vi "Alrebei.vi"() -> ()   [LabVIEW 2019]
panel:
  out "NH3/CH4":bool
  out "CH4":bool
  in  "Fuel Type":bool
  out "Waveform Chart":dbl(graph)
  out "time":dbl
  out "Controller":bool
  in  "PID gains":T1={"proportional gain (Kc)"=1.0, "integral time (Ti, min)"=0.01, "derivative time (Td, min)"=0.0} {"derivative time (Td, min)" format="%.3f"; "integral time (Ti, min)" format="%.3f"; "proportional gain (Kc)" format="%.3f"}
  in  "Fuel Control   (On/OFF)":bool=TRUE
  out "Controlled fuel\n       (kg/s)l":dbl
  out "Net Work (kW)":dbl(knob) scale=0.0..3000.0
  out "Turbine Work (kW)":dbl(knob) scale=0.0..3000.0
  out "Dilution Compressor Work (kW)":dbl(knob) scale=0.0..1000.0
  out "?":dbl(knob) scale=0.0..1000.0
  out "Dilution Compressor Work (kJ/Kg)":dbl(knob) scale=0.0..1000.0
  out "Flue gas  (kg/s)":dbl
  out "Comb. total (kg/s)":dbl(slide)
  out "?":dbl(slide) scale=0.0..2.5
  out "Comb. Air (kg/s)":dbl
  out "?":bool
  in  "Dilution Air (kg/s)":dbl(slide) scale=0.0..4.0
  out "?":bool
  out "?":bool
  out "?":bool
  out "?":bool
  out "Dilution Graphics.":bool
  out "?":dbl(slide)
  out "?":dbl(slide) scale=0.0..4.2
  out "Stoic. Condition":dbl
  out "?":dbl(slide)
  out "Comp. Air outlet Graphics":dbl(slide) scale=0.0..2.5
  out "?":dbl(slide)
  out "Fuel Graphics":dbl(slide) scale=0.0..0.14
  out "?":dbl(slide)
  out "?":dbl(slide) scale=0.0..0.14
  in  "Primery Air (kg/s)":dbl(slide) scale=1.0..4.0
  in  "Fuel (kg/s)":dbl(slide) scale=0.0..0.14
  out "?":dbl(slide)
  out "Primery Air  Graphics":dbl(slide) scale=0.0..4.0
  in  "Turbi. Eff.":dbl
  out "Turbine Outlet Prs.  (bar)":dbl(knob) scale=0.0..10.0
  out "Turbine Outlet Temp.  (K)":dbl(slide) scale=0.0..2000.0
  out "Turbine Work (kJ/kg)":dbl(knob) scale=0.0..3000.0
  out "Primery Compressor Work  (kJ/kg)      Primery Compressor Work ( kW)":dbl(knob) scale=0.0..1000.0
  in  "compressor \nefficiency":dbl
  out "ON/OFF":bool
  in  "RUN":bool
  out "Net Work (kJ/kg)":dbl(knob) scale=0.0..3000.0
  in  "Turbine Pres. ratio":dbl(slide) scale=0.0..1.0
  in  "Comp. Pres. ratio":dbl(slide) scale=0.0..10.0
  in  "Compressor\nTemp.":dbl(slide) scale=0.0..800.0
  in  "Compressor  Inlet Pressure  (bar)":dbl(knob) scale=0.0..3.0
  out "Turbine Inlet Temp. (K)":dbl(slide) scale=0.0..2000.0
  out "Turbine Inlet Pressure.\n               (bar)":dbl(knob) scale=0.0..10.0
  out "Compressor outlet Temp. (K)":dbl(slide) scale=0.0..1500.0
  out "Compressor outlet  pressure (bar)":dbl(knob) scale=0.0..10.0
  out "FUEL REDUCTION IS REQUIRED":bool
  out "DILUATION IS REQUIRED":bool
  out "Action Required":string
  out "COOLING IS ENOUGH":bool
  in  "Min T(K)":dbl
  in  "Max T (K)":dbl
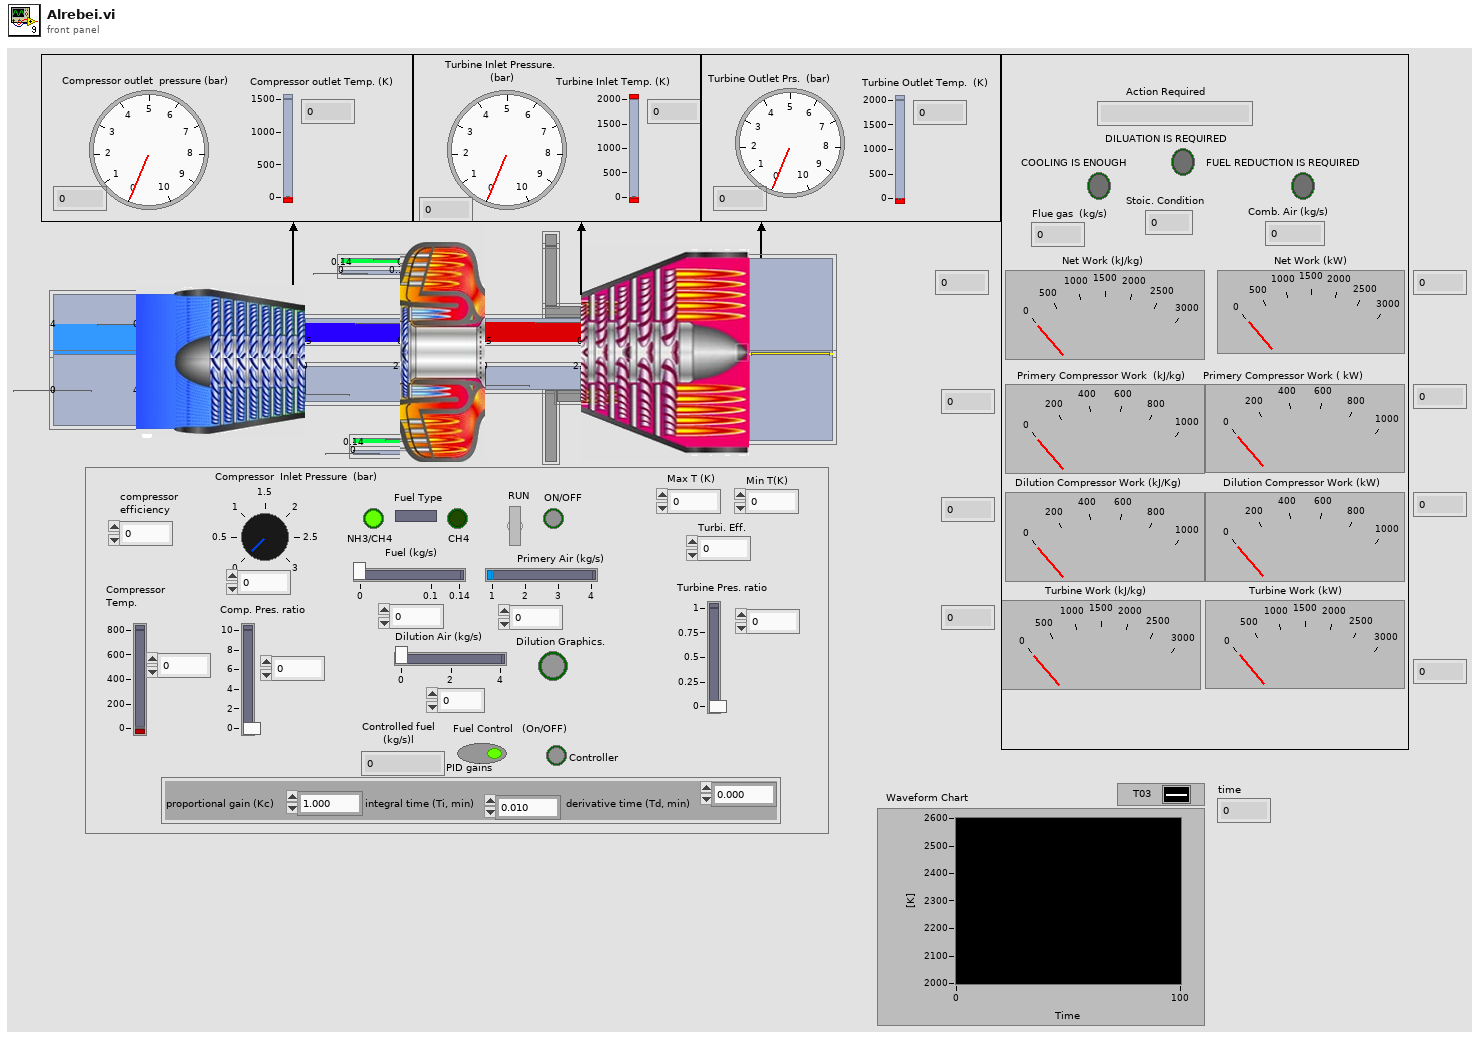
[diagram p1: front panel]
types:
  T1 = cluster{"proportional gain (Kc)":dbl, "integral time (Ti, min)":dbl, "derivative time (Td, min)":dbl}
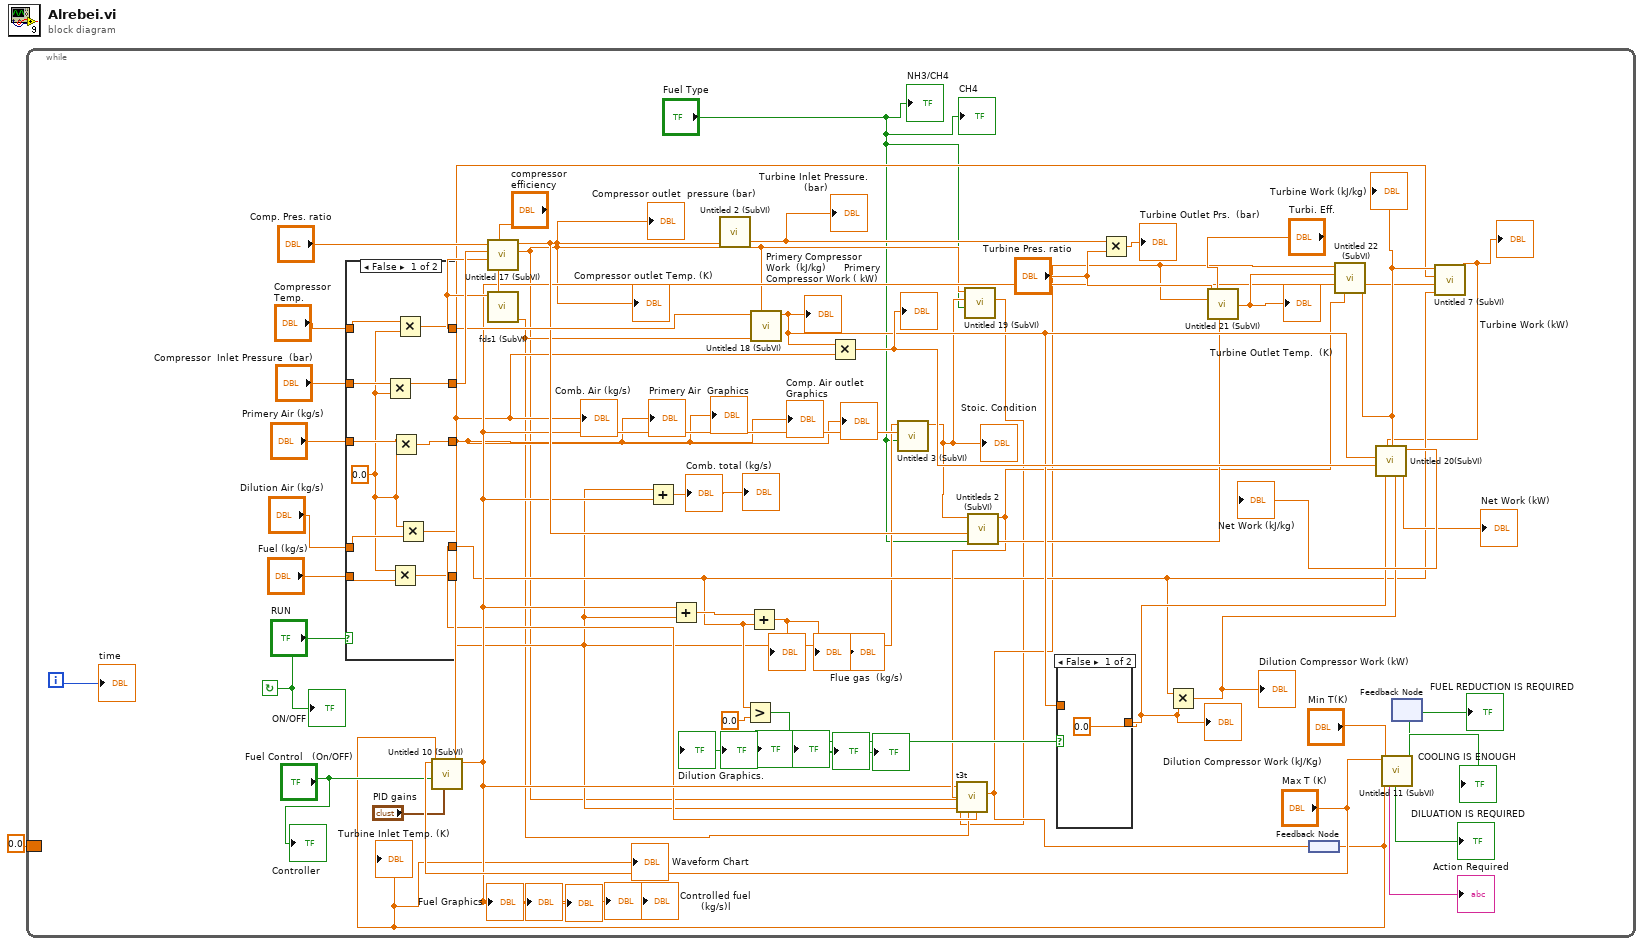
[diagram p0: block diagram]
diagram:
  n1 = while {
    border: 0.0 -> [_]
    i -> [w9]
    stop <- "RUN" continue-if-true
    n2 = case shown="False" "RUN" {
      tunnel: [w64 w71] -> w30
      tunnel: [w65 w72] -> w12
      tunnel: "Primery Air (kg/s)" -> [w67 w72]
      tunnel: "Fuel (kg/s)" -> [w66 w71]
      tunnel: [w62 w70] -> w13
      tunnel: "Dilution Air (kg/s)" -> [w63 w70]
      tunnel: [w60 w69] -> w39
      tunnel: "Compressor  Inlet Pressure  (bar)" -> [w61 w69]
      tunnel: [w58 w68] -> w21
      tunnel: "Compressor\nTemp." -> [w59 w68]
      frame False {
        w57 = 0.0
        n3 = Multiply(x=w61, y=w57) -> (x*y=w60:dbl)
        n4 = Multiply(x=w57, y=w66) -> (x*y=w64:dbl)
        n5 = Multiply(x=w67, y=w57) -> (x*y=w65:dbl)
        n6 = Multiply(x=w59, y=w57) -> (x*y=w58:dbl)
        n7 = Multiply(x=w57, y=w63) -> (x*y=w62:dbl)
      }
      frame True {
      }
    }
    "Primery Air  Graphics" <- w12
    "?" <- w12
    "Comp. Air outlet Graphics" <- w12
    "?" <- w12
    "Comb. Air (kg/s)" <- w12
    n8 = call "fds1 (SubVI).vi"("Compressor\nTemp."=w21) -> ("cpair"=w10:dbl, "gammair"=w20:dbl)  [unwired: 9 in]
    n9 = call "Untitled 17 (SubVI).vi"("Comp. Eff"="compressor \nefficiency", "gammaair"=w20, "Compressor inlet Tempreture (K)"=w21, "Compressor Inlet Pressure (bar)"=w39, "Compressor pressure ratio"="Comp. Pres. ratio") -> ("Compressor outlet Temp. (K)"=w6:dbl, "Compressor outlet Prs. (bar)"=w19:dbl)  [unwired: 5 in]
    "Compressor outlet  pressure (bar)" <- w19
    "Compressor outlet Temp. (K)" <- w6
    n10 = call "Untitled 2 (SubVI).vi"("Numeric in"=w19) -> ("Numeric out"=w48:dbl)  [unwired: 10 in]
    "Turbine Inlet Pressure.\n               (bar)" <- w48
    n11 = Greater?(x=w13, y=0.0) -> (0:w24:bool)
    "Dilution Graphics." <- w24
    "?" <- w24
    "?" <- w24
    "?" <- w24
    "?" <- w24
    "?" <- w24
    n12 = call "Untitled 18 (SubVI).vi"("Cpair"=w10, "Numeric in"=w6, "Compressor inlet Tempreture (K)"=w21) -> ("Numeric out"=w25:dbl)  [unwired: 8 in]
    "Primery Compressor Work  (kJ/kg)      Primery Compressor Work ( kW)" <- w25
    n13 = Multiply(x=w25, y=w12) -> (x*y=w33:dbl)
    "?" <- w33
    n14 = case shown="False" w24 {
      tunnel: w25 -> [_ w56]
      tunnel: [0.0 w56] -> w22
      frame False {
      }
      frame True {
      }
    }
    "Dilution Compressor Work (kJ/Kg)" <- w22
    n15 = Multiply(x=w48, y="Turbine Pres. ratio") -> (x*y=→"Turbine Outlet Prs.  (bar)":dbl)
    n16 = Multiply(x=w13, y=w22) -> (x*y=w34:dbl)
    "Dilution Compressor Work (kW)" <- w34
    n17 = feedback #1() -> (w8:dbl)
    "Turbine Inlet Temp. (K)" <- w8
    "Waveform Chart" <- w8
    n18 = call "Untitled 10 (SubVI).vi"("Fuel (kg/s)"=w30, "PID gains"="PID gains", "Fuel Control   (On/OFF)"="Fuel Control   (On/OFF)", "Numeric"=w8, "Max T (K)"="Max T (K)") -> ("output"=w14:dbl)  [unwired: 6 in]
    "?" <- w14
    "?" <- w14
    "Fuel Graphics" <- w14
    "?" <- w14
    "Controlled fuel\n       (kg/s)l" <- w14
    n19 = Add(x=w12, y=w14) -> (x+y=→"?" →"Comb. total (kg/s)":dbl)
    n20 = Add(x=w14, y=w12) -> (x+y=w16:dbl)
    n21 = Add(x=w16, y=w13) -> (x+y=→"?" →"?" →"Flue gas  (kg/s)":dbl)
    n22 = call "Untitled 3 (SubVI).vi"("Fuel Type"="Fuel Type", "Fuel (kg/s)"=w14, "Primery Air (kg/s)"=w12) -> ("Stoic"=w5:dbl)  [unwired: 8 in]
    "Stoic. Condition" <- w5
    n23 = call "Untitled 19 (SubVI).vi"("Fuel type"="Fuel Type", "Stoic condition"=w5, "T02"=w6) -> ("T03"=w3:dbl)  [unwired: 8 in]
    n24 = call "Untitleds 2 (SubVI).vi"("Fuel Type"="Fuel Type", "T2"=w19, "stoic"=w5) -> ("gamma g"=w18:dbl, "cpg"=w17:dbl)  [unwired: 7 in]
    n25 = call "t3t.vi"("T2"=w6, "fuel (kg/s)"=w14, "cpg"=w17, "T3"=w3, "cpa"=w10, "Primery Air (kg/s)"=w12, "Dilution Air (kg/s)"=w13) -> ("T03t"=w4:dbl)  [unwired: 3 in]
    n26 = call "Untitled 21 (SubVI).vi"("gammag"=w18, "Turbi. Eff."="Turbi. Eff.", "T3t"=w4, "Turbine prssure ratio"="Turbine Pres. ratio") -> ("T4"=w44:dbl)  [unwired: 7 in]
    "Turbine Outlet Temp.  (K)" <- w44
    n27 = feedback-in #1(w4) -> ()
    n28 = call "Untitled 22 (SubVI).vi"("cpg"=w17, "t4"=w44, "t3t"=w4) -> ("wt"=w15:dbl)  [unwired: 8 in]
    "Turbine Work (kJ/kg)" <- w15
    n29 = call "Untitled 11 (SubVI).vi"("Recorded T (K)"=w8, "Min T(K)"="Min T(K)", "Max T (K)"="Max T (K)") -> ("SHUTDOWN IS REQUIRED"=w32:bool, "DILUATION IS REQUIRED"=→"DILUATION IS REQUIRED":bool, "COOLING IS ENOUGH"=→"COOLING IS ENOUGH":bool, "String"=→"Action Required":string)  [unwired: 5 in]
    n30 = feedback-in #2(w32) -> ()
    n31 = feedback #2() -> (→"FUEL REDUCTION IS REQUIRED":bool)  [unwired: 1 in]
    n32 = call "Untitled 7 (SubVI).vi"("dilution"=w13, "fuel"=w14, "primery air"=w12, "w_t_dot"=w15) -> ("wt"=w11:dbl)  [unwired: 7 in]
    "Turbine Work (kW)" <- w11
    n33 = call "Untitled 20(SubVI).vi"("Numeric 2"=w34, "Numeric out 3"=w22, 7:"Numeric in"=w11, "Numeric"=w33, 10:"Numeric in"=w25, "Numeric 4"=w15) -> ("Numeric 3"=→"Net Work (kW)":dbl, "Numeric 5"=→"Net Work (kJ/kg)":dbl)  [unwired: 4 in]
    "ON/OFF" <- "RUN"
    "Controller" <- "Fuel Control   (On/OFF)"
    "time" <- w9
    "CH4" <- "Fuel Type"
    "NH3/CH4" <- "Fuel Type"
  }
